vi "Read System Information.vi"(8 "Error in":errorcluster caption="错误输入", 10 "Channel":dbl caption="设备通道", 11 "Modbus master in":refnum<class "Modbus Master.lvclass"> caption="Modbus实例输入") -> (0 "Error out":errorcluster caption="错误输出", 1 "Hardware Revision":string caption="硬件版本", 2 "Serial Number":string caption="序 列 号", 3 "Modbus instance out":refnum<class "Modbus API.lvclass"> caption="Modbus实例输出", 4 "Firmware Revision":string caption="固件版本", 5 "Model Number":string caption="设备型号")   [LabVIEW 2023, in "Longer Pump dLSP501 Series.lvlib"]
doc: "读取系统信息。包括：设备型号、序列号、硬件版本、固件版本。"
uses:
  <instrlib>/Longer Pump dLSP501 Modbus RTU Series/Longer Pump dLSP501 Series.lvlib
  <vilib>/NI/Modbus Library/API/Modbus API.lvclass
  <vilib>/NI/Modbus Library/API/Master/Modbus Master.lvclass
  C:/Program Files/National Instruments/LabVIEW 2023/vi.lib/NI/Modbus Library/API/Modbus API.lvclass
  <vilib>/Utility/miscctls.llb/LVFontTypeDef.ctl
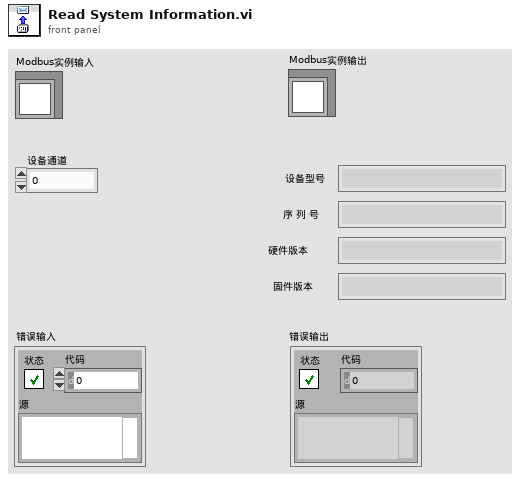
[diagram p1: front panel]
types:
  T1 = typedef "LVFontTypeDef.ctl" = cluster{"Font Name":string, "Size":u16, "Bold":bool, "Italic":bool, "Underline":bool, "Strikeout":bool, "Color":u32}
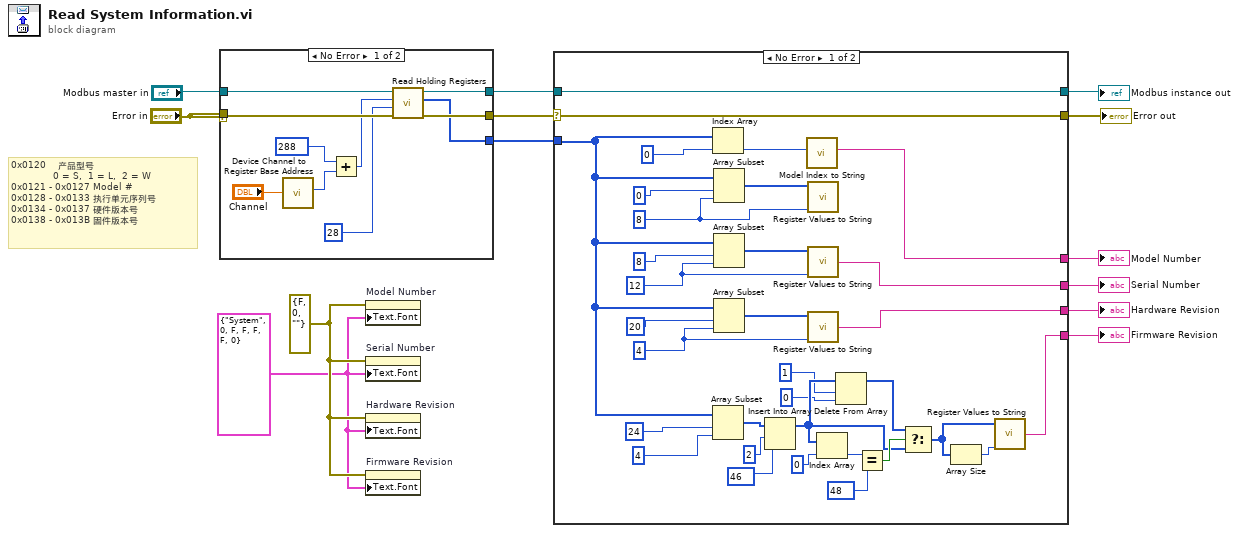
[diagram p0: block diagram]
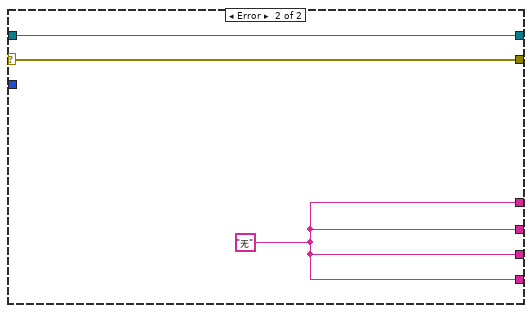
[diagram p2: hidden frame]
diagram:
  w4 = errorcluster {"status"=FALSE, "code"=0, "source"=""} ("错误输入（无错误）")
  w3 = T1 {"Font Name"="System", "Size"=0, "Bold"=FALSE, "Italic"=FALSE, "Underline"=FALSE, "Strikeout"=FALSE, "Color"=0} ("文本.字体")
  # "0x0120\t   产品型号\n              0 = S,  1 = L,  2 = W\n0x0121 - 0x0127\tModel #\n0x0128 - 0x0133\t执行单元序列号\n0x0134 - 0x0137\t硬件版本号\n0x0138 - 0x013B\t固件版本号"
  n1 = case shown="No Error" "Error in" {
    selector: "Error in" -> [_ w25]
    tunnel: "Error in" -> [w23 _]
    tunnel: [w22 w25] -> w12
    tunnel: [w21 w24] -> w11
    tunnel: "Modbus master in" -> [w20 w24]
    tunnel: [w18 _] -> w9
    frame No Error {
      n2 = call <instrlib>:"Device Channel to Register Base Address.vi"("Channel"="Channel") -> ("Register Base Address"=w16:u16)  [unwired: 10 in]
      n3 = Add(x=u16 288 ("address"), y=w16) -> (x+y=w14:u16)
      n4 = call-dynamic "Read Holding Registers.vi"("error in"=w23, "number of inputs"=u16 28 ("address"), "starting address"=w14, "Modbus master in"=w20) -> ("error out"=w22:errorcluster, "register values"=w18:u16[], "Modbus master out"=w21:refnum<class "Modbus Master.lvclass">)  [unwired: 5 in]
    }
    frame Error {
    }
  }
  n5 = property on="Model Number" class="Str"(error in=w4, "Text.Font"=w3) -> ()  [unwired: 1 in, 2 out]
  n6 = property on="Serial Number" class="Str"(error in=w4, "Text.Font"=w3) -> ()  [unwired: 1 in, 2 out]
  n7 = property on="Hardware Revision" class="Str"(error in=w4, "Text.Font"=w3) -> ()  [unwired: 1 in, 2 out]
  n8 = property on="Firmware Revision" class="Str"(error in=w4, "Text.Font"=w3) -> ()  [unwired: 1 in, 2 out]
  n9 = case shown="No Error" w12 {
    selector: w12 -> [w57 w60]
    tunnel: w11 -> [w58 w61]
    tunnel: [w58 w61] -> w10
    tunnel: [w57 w60] -> w2
    tunnel: [w50 w59] -> w5
    tunnel: w9 -> [w41 _]
    tunnel: [w51 w59] -> w8
    tunnel: [w39 w59] -> w7
    tunnel: [w49 w59] -> w6
    frame No Error {
      w44 = u16 4 ("address")
      w45 = u16 12 ("address")
      w54 = u16 8 ("address")
      n10 = Index Array(array=w41, index=u16 0 ("元素")) -> (element=w40:u16)
      n11 = Array Subset(array=w41, index=u16 24 ("address"), length=u16 4 ("address")) -> (w38:u16[])
      n12 = Array Subset(array=w41, index=u16 0 ("address"), length=w54) -> (w55:u16[])
      n13 = Array Subset(array=w41, index=u16 8 ("address"), length=w45) -> (w53:u16[])
      n14 = Array Subset(array=w41, index=u16 20 ("address"), length=w44) -> (w52:u16[])
      n15 = Insert Into Array(array=w38, index=2 ("索引"), new element=u16 46 ("新元素/子数组")) -> (w31:u16[])
      n16 = call <instrlib>:"Model Index to String.vi"("Code"=w40) -> ("Info String"=w39:string)  [unwired: 10 in]
      n17 = call <instrlib>:"Register Values to String.vi"("Register Values"=w55, "Register Number"=w54) -> ()  [unwired: 5 in, 1 out]
      n18 = call <instrlib>:"Register Values to String.vi"("Register Values"=w53, "Register Number"=w45) -> ("String Out"=w51:string)  [unwired: 5 in]
      n19 = call <instrlib>:"Register Values to String.vi"("Register Values"=w52, "Register Number"=w44) -> ("String Out"=w50:string)  [unwired: 5 in]
      n20 = Index Array(array=w31, index=0 ("索引")) -> (element=w34:u16)
      n21 = Delete From Array(array=w31, length=1 ("长度"), index=0 ("索引")) -> (array with subset deleted=w28:u16[])  [unwired: 1 out]
      n22 = Equal?(x=w34, y=u16 48 ("新元素/子数组")) -> (x = y?=w32:bool)
      n23 = Select(t=w28, s=w32, f=w31) -> (s? t:f=w27:u16[])
      n24 = Array Size(array=w27) -> (size(s)=w26:i32)
      n25 = call <instrlib>:"Register Values to String.vi"("Register Values"=w27, "Register Number"=w26) -> ("String Out"=w49:string)  [unwired: 5 in]
    }
    frame Error {
      w59 = "无"
    }
  }
  "Modbus instance out" <- w10
  "Firmware Revision" <- w6
  "Model Number" <- w7
  "Serial Number" <- w8
  "Hardware Revision" <- w5
  "Error out" <- w2
